vi "DCMotor_PickMotorSelector.vi"(7 "DCMOTOR_TYPES":T1, 11 "Num Motors":i32=1) -> (3 "DCMOTOR":T2 {"Jr_KgM2" format="%13.5p"; "L_H" format="%13.5p"; "Kt_NMPerAmp" format="%13.5p"; "KvINV_RadPerSecPerVolt" format="%13.5p"; "R_Ohms" format="%13.5p"; "FreeSpeed_RadPerSec" format="%13.5p"; "FreeCurrent_Amps" format="%13.5p"; "StallCurrent_Amps" format="%13.5p"; "StallTorque_NM" format="%13.5p"; "nominalVoltage_Volts" format="%13.5p"})   [LabVIEW 2019, in "Trajectory_Library.lvlib"]
doc: "Creates a new DC MOTOR data cluster for a custom motor of the chosen type.. \n\nInputs: \n - DC Motor Type -- The model of the motor.\n - Num Motors -- The number of motors used together in this sytem driving the same load.\n\nOutputs:\n - DCMOTOR -- Cluster containing the motor modeling constants for this set of motors."
uses:
  Trajectory_Library.lvlib
  TypeDef/DCMOTOR.CTL
  Enum/DCMOTOR_TYPES_ENUM.ctl
  DCMotor_New.vi
  VI/Units_RotationsPerMinuteToRadiansPerSecond.vi
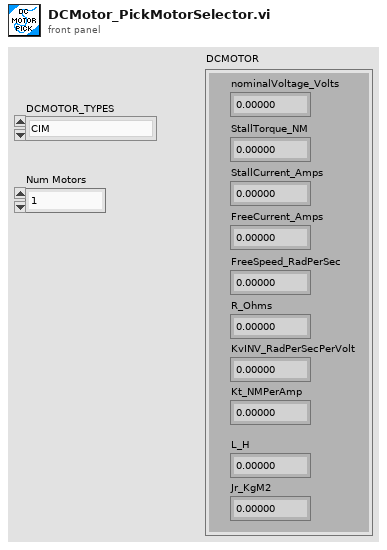
[diagram p1: front panel]
types:
  T1 = typedef "Trajectory_Library.lvlib/DCMOTOR_TYPES_ENUM.ctl" = enum16{"CIM", "AndyMark 9015", "Andy Mark RS 775 125", "Bag", "BaneBots RS 550", "BaneBots RS 775", "Falcon 500", "Mini CIM", "NEO", "NEO 550", "Romi BuiltIn", "Vex 775 Pro", "Snow Blower AM 2235A", "Bosch Seat AM 3493", "Falcon 500 FOC", "Kraken X60", "Kraken X60 FOC", "NEO Vortex", "Minion", "Kraken X44", "Kraken X44 FOC"}
  T2 = typedef "Trajectory_Library.lvlib/DCMOTOR.CTL" = cluster{"nominalVoltage_Volts":dbl, "StallTorque_NM":dbl, "StallCurrent_Amps":dbl, "FreeCurrent_Amps":dbl, "FreeSpeed_RadPerSec":dbl, "R_Ohms":dbl, "KvINV_RadPerSecPerVolt":dbl, "Kt_NMPerAmp":dbl, "L_H":dbl, "Jr_KgM2":dbl}
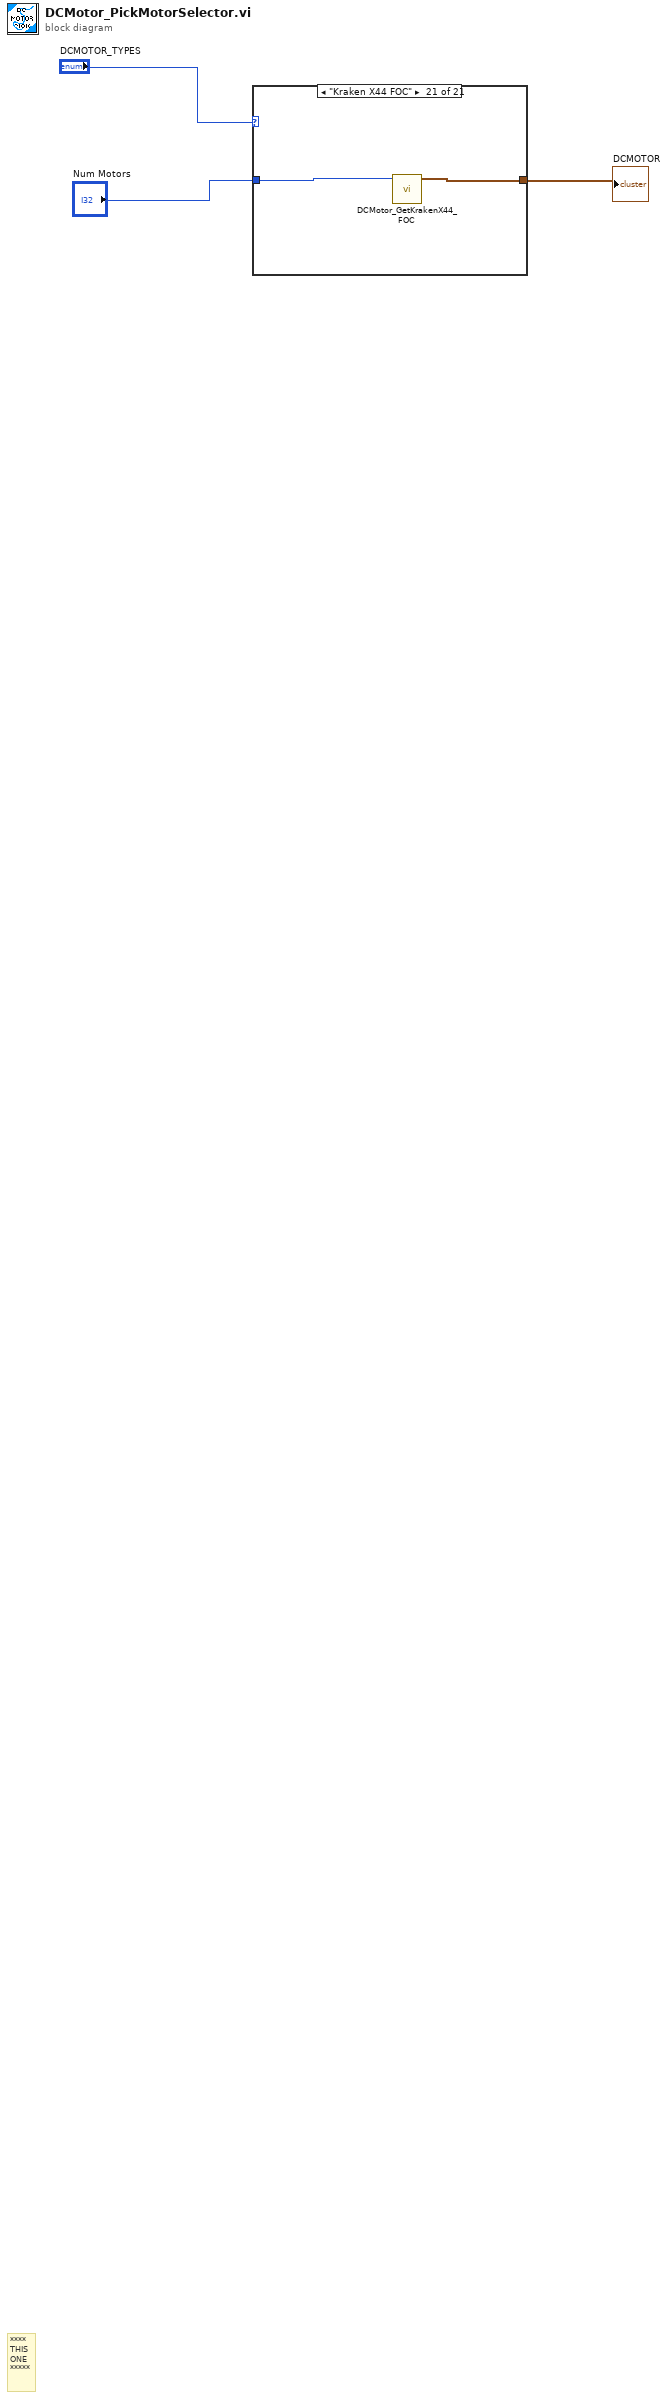
[diagram p0: block diagram]
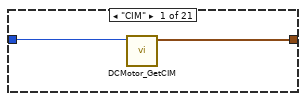
[diagram p2: hidden frame]
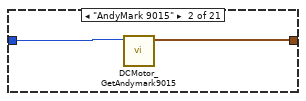
[diagram p3: hidden frame]
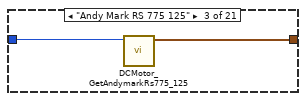
[diagram p4: hidden frame]
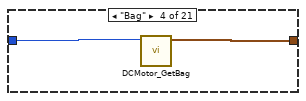
[diagram p5: hidden frame]
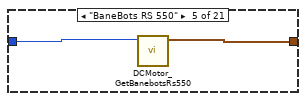
[diagram p6: hidden frame]
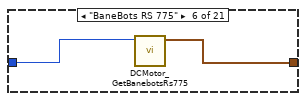
[diagram p7: hidden frame]
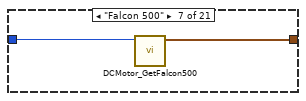
[diagram p8: hidden frame]
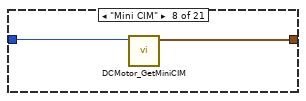
[diagram p9: hidden frame]
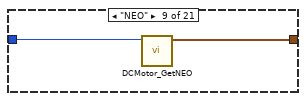
[diagram p10: hidden frame]
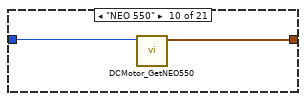
[diagram p11: hidden frame]
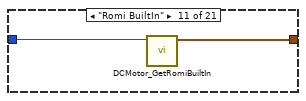
[diagram p12: hidden frame]
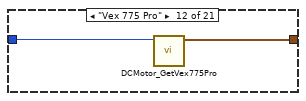
[diagram p13: hidden frame]
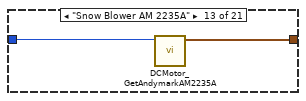
[diagram p14: hidden frame]
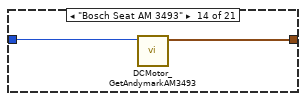
[diagram p15: hidden frame]
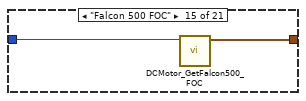
[diagram p16: hidden frame]
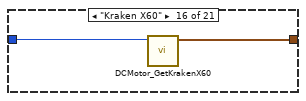
[diagram p17: hidden frame]
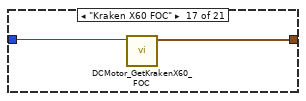
[diagram p18: hidden frame]
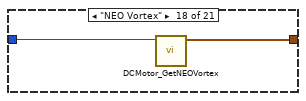
[diagram p19: hidden frame]
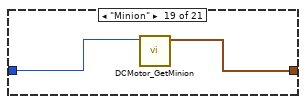
[diagram p20: hidden frame]
diagram:
  # "****\nTHIS\nONE\n*****"
  n1 = case shown="\"Kraken X44 FOC\"" "DCMOTOR_TYPES" {
    tunnel: [w5 w7 w9 w11 w13 w15 w17 w19 w21 w23 w25 w27 w29 w31 w33 w35 w37 w39 w40 w42 w44] -> w2
    tunnel: "Num Motors" -> [w4 w6 w8 w10 w12 w14 w16 w18 w20 w22 w24 w26 w28 w30 w32 w34 w36 w38 w41 w43 w45]
    frame "CIM" {
      n2 = call "DCMotor_GetCIM.vi"("Num Motors"=w4) -> ("DCMOTOR"=w5:T2)  [unwired: 10 in]
    }
    frame "AndyMark 9015" {
      n3 = call "DCMotor_GetAndymark9015.vi"("Num Motors"=w6) -> ("DCMOTOR"=w7:T2)  [unwired: 10 in]
    }
    frame "Andy Mark RS 775 125" {
      n4 = call "DCMotor_GetAndymarkRs775_125.vi"("Num Motors"=w8) -> ("DCMOTOR"=w9:T2)  [unwired: 10 in]
    }
    frame "Bag" {
      n5 = call "DCMotor_GetBag.vi"("Num Motors"=w10) -> ("DCMOTOR"=w11:T2)  [unwired: 10 in]
    }
    frame "BaneBots RS 550" {
      n6 = call "DCMotor_GetBanebotsRs550.vi"("Num Motors"=w12) -> ("DCMOTOR"=w13:T2)  [unwired: 10 in]
    }
    frame "BaneBots RS 775" {
      n7 = call "DCMotor_GetBanebotsRs775.vi"("Num Motors"=w14) -> ("DCMOTOR"=w15:T2)  [unwired: 10 in]
    }
    frame "Falcon 500" {
      n8 = call "DCMotor_GetFalcon500.vi"("Num Motors"=w16) -> ("DCMOTOR"=w17:T2)  [unwired: 10 in]
    }
    frame "Mini CIM" {
      n9 = call "DCMotor_GetMiniCIM.vi"("Num Motors"=w18) -> ("DCMOTOR"=w19:T2)  [unwired: 10 in]
    }
    frame "NEO" {
      n10 = call "DCMotor_GetNEO.vi"("Num Motors"=w20) -> ("DCMOTOR"=w21:T2)  [unwired: 10 in]
    }
    frame "NEO 550" {
      n11 = call "DCMotor_GetNEO550.vi"("Num Motors"=w22) -> ("DCMOTOR"=w23:T2)  [unwired: 10 in]
    }
    frame "Romi BuiltIn" {
      n12 = call "DCMotor_GetRomiBuiltIn.vi"("Num Motors"=w24) -> ("DCMOTOR"=w25:T2)  [unwired: 10 in]
    }
    frame "Vex 775 Pro" {
      n13 = call "DCMotor_GetVex775Pro.vi"("Num Motors"=w26) -> ("DCMOTOR"=w27:T2)  [unwired: 10 in]
    }
    frame "Snow Blower AM 2235A" {
      n14 = call "DCMotor_GetAndymarkAM2235A.vi"("Num Motors"=w28) -> ("DCMOTOR"=w29:T2)  [unwired: 10 in]
    }
    frame "Bosch Seat AM 3493" {
      n15 = call "DCMotor_GetAndymarkAM3493.vi"("Num Motors"=w30) -> ("DCMOTOR"=w31:T2)  [unwired: 10 in]
    }
    frame "Falcon 500 FOC" {
      n16 = call "DCMotor_GetFalcon500_FOC.vi"("Num Motors"=w32) -> ("DCMOTOR"=w33:T2)  [unwired: 10 in]
    }
    frame "Kraken X60" {
      n17 = call "DCMotor_GetKrakenX60.vi"("Num Motors"=w34) -> ("DCMOTOR"=w35:T2)  [unwired: 10 in]
    }
    frame "Kraken X60 FOC" {
      n18 = call "DCMotor_GetKrakenX60_FOC.vi"("Num Motors"=w36) -> ("DCMOTOR"=w37:T2)  [unwired: 10 in]
    }
    frame "NEO Vortex" {
      n19 = call "DCMotor_GetNEOVortex.vi"("Num Motors"=w38) -> ("DCMOTOR"=w39:T2)  [unwired: 10 in]
    }
    frame "Minion" {
      n20 = call "DCMotor_GetMinion.vi"("Num Motors"=w41) -> ("DCMOTOR"=w40:T2)  [unwired: 10 in]
    }
    frame "Kraken X44" {
      n21 = call "DCMotor_GetKrakenX44.vi"("Num Motors"=w43) -> ("DCMOTOR"=w42:T2)  [unwired: 10 in]
    }
    frame "Kraken X44 FOC" {
      n22 = call "DCMotor_GetKrakenX44_FOC.vi"("Num Motors"=w45) -> ("DCMOTOR"=w44:T2)  [unwired: 10 in]
    }
  }
  "DCMOTOR" <- w2
